vi "DPO_7K_AcquireChannels.vi"(8 "Error In":errorcluster, 10 "Settings":T3={"Channels to acquire"=[0, 1, 2, 3], "Bandwidth"=0, "#Avg"=0, "Trigger Channel"=0, "Trigger Level"=0.0, "Sampling Frequency"=0, "Epoch"=0.0, "Enable Autoscale?"=FALSE} {"Bandwidth" items=["500 MHz", "1 GHz", "2 GHz", "3 GHz", "4 GHz", "5 GHz", "6 GHz", "7 GHz", "8 GHz", "9 GHz", "10 GHz", "11 GHz", "12 GHz", "13 GHz", "14 GHz", "15 GHz", "16 GHz", "17 GHz", "18 GHz", "19 GHz", "20 GHz", "21 GHz", "22 GHz", "23 GHz", "24 GHz", "25 GHz", "26 GHz", "27 GHz", "28 GHz", "29 GHz", "30 GHz", "31 GHz", "32 GHz", "33 GHz", "33 GHz HW (Tek)", "34 GHz (ATI)", "35 GHz (ATI)", "36 GHz (ATI)", "38 GHz (ATI)", "40 GHz (ATI)", "45 GHz (ATI)", "50 GHz (ATI)"]; "Epoch" format="%#_6ps"; "Sampling Frequency" items=["3.125 Sa/s", "5 Sa/s", "6.25 Sa/s", "7.8125 Sa/s", "10 Sa/s", "12.5 Sa/s", "15.625 Sa/s", "20 Sa/s", "25 Sa/s", "31.25 Sa/s", "50 Sa/s", "62.5 Sa/s", "78.125 Sa/s", "100 Sa/s", "125 Sa/s", "156.25 Sa/s", "200 Sa/s", "250 Sa/s", "312.5 Sa/s", "390.625 Sa/s", "400 Sa/s", "500 Sa/s", "625 Sa/s", "781.25 Sa/s", "1 kSa/s", "1.25 kSa/s", "1.5625 kSa/s", "2 kSa/s", "2.5 kSa/s", "3.125 kSa/s", "3.90625 kSa/s", "4 kSa/s", "5 kSa/s", "6.25 kSa/s", "7.8125 kSa/s", "10 kSa/s", "12.5 kSa/s", "15.625 kSa/s", "20 kSa/s", "25 kSa/s", "31.25 kSa/s", "39.0625 kSa/s", "50 kSa/s", "62.5 kSa/s", "78.125 kSa/s", "100 kSa/s", "125 kSa/s", "156.25 kSa/s", "200 kSa/s", "244.14063 kSa/s", "250 kSa/s", "312.5 kSa/s", "390.625 kSa/s", "500 kSa/s", "625 kSa/s", "781.25 kSa/s", "1 MSa/s", "1.2207 MSa/s", "1.25 MSa/s", "1.5625 MSa/s", "1.95313 MSa/s", "2.44141 MSa/s", "2.5 MSa/s", "3.125 MSa/s", "3.90625 MSa/s", "4.88281 MSa/s", "5 MSa/s", "6.25 MSa/s", "7.8125 MSa/s", "9.76563 MSa/s", "12.5 MSa/s", "1.5625 MSa/s", "25 MSa/s", "31.25 MSa/s", "39.0625 MSa/s", "62.5 MSa/s", "78.125 MSa/s", "125 MSa/s", "156.25 MSa/s", "250 MSa/s", "312.5 MSa/s", "625 MSa/s", "781.25 MSa/s", "1.25 GSa/s", "1.5625 GSa/s", "3.125 GSa/s", "6.25 GSa/s", "12.5 GSa/s", "25 GSa/s", "50 GSa/s", "100 GSa/s", "200 GSa/s (ATI only)"]; "Trigger Channel" items=["Channel 1", "Channel 2", "Channel 3", "Channel 4", "Auxiliary", "Line"]; "Channels to acquire" items=["Channel 1", "Channel 2", "Channel 3", "Channel 4", "Math 1", "Math 2", "Math 3", "Math 4", "Reference 1", "Reference 2", "Reference 3", "Reference 4"]}, 11 "VISA Resource Name In":refnum<visa-resource-name>) -> (0 "Error Out":errorcluster, 2 "Acquired Data":waveform(dbl)[](array[waveform]), 3 "VISA Resource Name Out":refnum<visa-resource-name>)   [LabVIEW 2020]
uses:
  DPO 7k Settings.ctl
  subVI/Return_To_Interface.ctl
  subVI/Set_Configuration.ctl
panel:
  out "Stop":bool
  in  "Set":T1
  in  "Return to Interface":T2
  # "ACQUIRE CHANNELS"
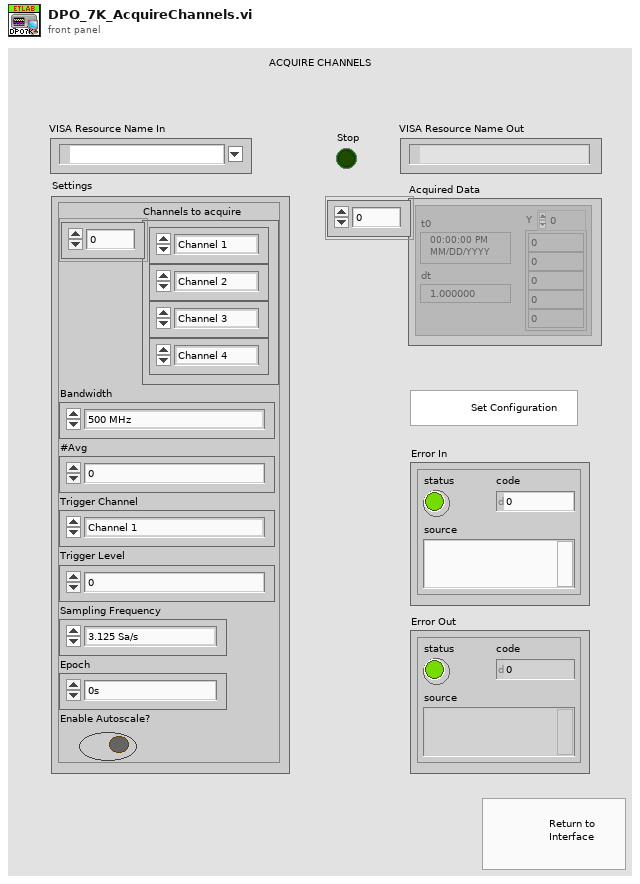
[diagram p1: front panel]
types:
  T1 = typedef "Set_Configuration.ctl" = bool
  T2 = typedef "Return_To_Interface.ctl" = bool
  T3 = typedef "DPO 7k Settings.ctl" = cluster{"Channels to acquire":u16[], "Bandwidth":u16, "#Avg":i32, "Trigger Channel":u16, "Trigger Level":dbl, "Sampling Frequency":u16, "Epoch":dbl, "Enable Autoscale?":bool}
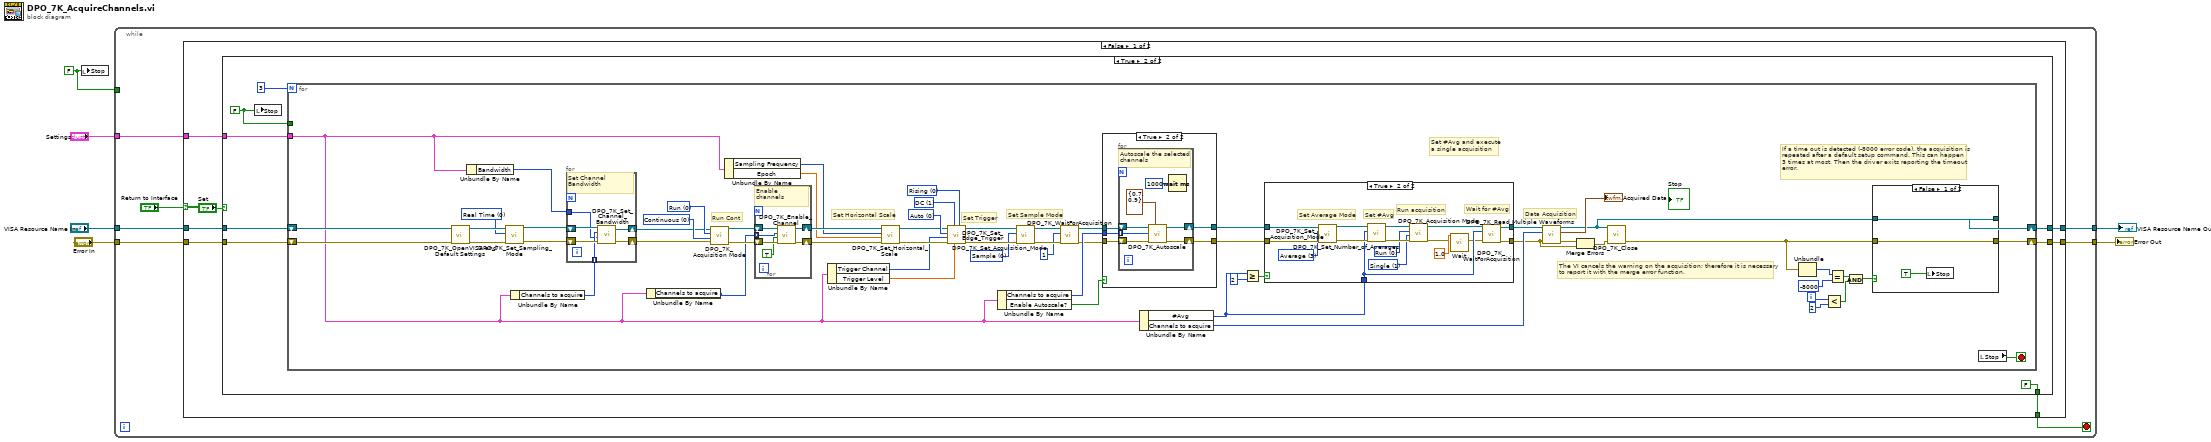
[diagram p0: block diagram]
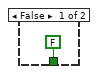
[diagram p2: hidden frame]
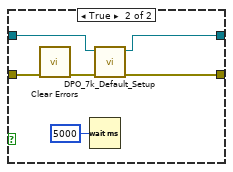
[diagram p3: hidden frame]
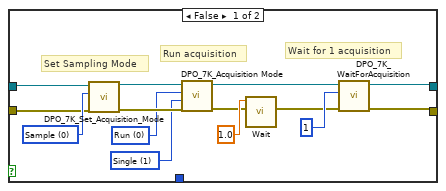
[diagram p4: hidden frame]
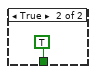
[diagram p6: hidden frame]
diagram:
  w1 = FALSE ("Stop")
  n1 = local write "Stop"(w1) -> ()
  n2 = while {
    tunnel: "Settings" -> [w9]
    tunnel: "VISA Resource Name In" -> [w12]
    tunnel: [w10] -> w3
    tunnel: "Error In" -> [w13]
    tunnel: [w11] -> w4
    tunnel: w1 -> [_]
    stop <- w7 stop-if-true
    n3 = case shown="False" "Return to Interface" {
      tunnel: w13 -> [w20 _]
      tunnel: w12 -> [w19 _]
      tunnel: [w18 _] -> w11
      tunnel: [w17 _] -> w10
      tunnel: w9 -> [w16 _]
      tunnel: [w14 TRUE] -> w7
      frame False {
        n4 = case shown="True" "Set" {
          tunnel: w20 -> [_ w29]
          tunnel: w19 -> [_ w28]
          tunnel: [_ w27] -> w18
          tunnel: [_ w26] -> w17
          tunnel: w16 -> [_ w25]
          tunnel: [FALSE FALSE] -> w14
          frame False {
          }
          frame True {
            w23 = FALSE
            n5 = local write "Stop"(w23) -> ()
            n6 = for {
              N: 3 -> [_]
              tunnel: w25 -> [w88]
              shift-right: [w86] -> w27
              shift-left: w29 -> [w90]
              shift-right: [w85] -> w26
              shift-left: w28 -> [w89]
              tunnel: w23 -> [_]
              i -> [w87]
              stop <- w30 stop-if-true
              w64 = u16 0 items=["Real Time", "Equivalent Time", "Interpolation"] ("Sampling Mode")
              w67 = u16 0 items=["Continuous", "Single"] ("Mode")
              w68 = u16 0 items=["Run", "Stop"] ("Action")
              w74 = u16 0 items=["Sample", "Peak Detect", "High resolution", "Average", "WFMDB", "Envelope"] ("Acquisition Mode")
              w82 = u16 0 items=["Auto", "Normal"] ("Trigger Mode")
              w83 = u16 1 items=["AC", "DC", "HF Reject (>50 kHz)", "LF Reject (<80 kHz)", "Noise Reject"] ("Trigger Coupling")
              w84 = u16 0 items=["Rising", "Falling", "Either"] ("Trigger Slope")
              # "If a time out is detected (-8000 error code), the acquisition is\nrepeated after a default setup command. This can happen\n3 times at most. Then the driver exits reporting the timeout\nerror."
              # "The VI cancels the warning on the acquisition; therefore it is necessary\nto report it with the merge error function."
              # "Set #Avg and execute\na single acquisition"
              # "Run Cont"
              # "Data Acquisition"
              # "Set Sample Mode"
              # "Set Trigger"
              # "Set Horizontal Scale"
              n7 = call "DPO_7K_OpenVISA and Default Settings.vi"("Error In"=w90, "VISA resource name in"=w89) -> ("error out"=w65:errorcluster, "VISA resource name out"=w66:refnum<visa-resource-name>)  [unwired: 8 in]
              n8 = Unbundle By Name(w88) -> ("Bandwidth"=w59:u16)
              n9 = call "DPO_7K_Set_Sampling_Mode.vi"("Error In"=w65, "Sampling Mode"=w64, "VISA resource name in"=w66) -> ("Error Out"=w62:errorcluster, "VISA resource name out"=w63:refnum<visa-resource-name>)  [unwired: 7 in]
              n10 = Unbundle By Name(w88) -> ("Channels to acquire"=w56:u16[])
              n11 = for {
                shift-right: [w146] -> w60
                shift-left: w63 -> [w149]
                shift-right: [w147] -> w61
                shift-left: w62 -> [w148]
                tunnel: w56 -> [w145] mode=indexing
                tunnel: w59 -> [w144]
                # "Set Channel Bandwidth"
                n12 = call "DPO_7K_Set_Channel_Bandwidth.vi"("Error In"=w148, "Bandwidth"=w144, "Channel"=w145, "VISA resource name in"=w149) -> ("Error Out"=w147:errorcluster, "VISA resource name out"=w146:refnum<visa-resource-name>)  [unwired: 6 in]
              }
              n13 = Unbundle By Name(w88) -> ("Channels to acquire"=w53:u16[])
              n14 = call "DPO_7K_Acquisition Mode.vi"("Error In"=w61, "Mode"=w67, "Action"=w68, "VISA resource name in"=w60) -> ("Error Out"=w70:errorcluster, "VISA resource name out"=w69:refnum<visa-resource-name>)  [unwired: 6 in]
              n15 = Unbundle By Name(w88) -> ("Sampling Frequency"=w58:u16, "Epoch"=w57:dbl)
              n16 = for {
                shift-right: [w154] -> w77
                shift-left: w70 -> [w153]
                shift-right: [w155] -> w78
                shift-left: w69 -> [w152]
                tunnel: w53 -> [w151] mode=indexing
                # "Enable\nchannels"
                n17 = call "DPO_7K_Enable_Channel.vi"("Error In"=w153, "Activate?"=TRUE, "Channel"=w151, "VISA resource name in"=w152) -> ("Error Out"=w154:errorcluster, "VISA resource name out"=w155:refnum<visa-resource-name>)  [unwired: 5 in, 1 out]
              }
              n18 = Unbundle By Name(w88) -> ("Trigger Channel"=w54:u16, "Trigger Level"=w55:dbl)
              n19 = call "DPO_7K_Set_Horizontal_Scale.vi"("Error In"=w77, "Epoch"=w57, "Sampling Frequency"=w58, "VISA resource name in"=w78) -> ("Error Out"=w80:errorcluster, "VISA resource name out"=w79:refnum<visa-resource-name>)  [unwired: 6 in]
              n20 = call "DPO_7K_Set_Edge_Trigger.vi"("Trigger Slope"=w84, "Trigger Level"=w55, "Trigger Coupling"=w83, "Error In"=w80, "Trigger Channel"=w54, "Trigger Mode"=w82, "VISA resource name in"=w79) -> ("Error Out"=w75:errorcluster, "VISA resource name out"=w76:refnum<visa-resource-name>)  [unwired: 3 in]
              n21 = Unbundle By Name(w88) -> ("Channels to acquire"=w52:u16[], "Enable Autoscale?"=w50:bool)
              n22 = call "DPO_7K_Set_Acquisition_Mode.vi"("Error In"=w75, "Acquisition Mode"=w74, "VISA resource name in"=w76) -> ("Error Out"=w42:errorcluster, "VISA resource name out"=w43:refnum<visa-resource-name>)  [unwired: 7 in]
              n23 = call "DPO_7K_WaitForAcquisition.vi"("Error In"=w42, "Number of Waveforms"=1, "VISA resource name in"=w43) -> ("Error Out"=w41:errorcluster, "VISA resource name out"=w40:refnum<visa-resource-name>)  [unwired: 7 in]
              n24 = case shown="True" w50 {
                tunnel: w40 -> [w131 w136]
                tunnel: w41 -> [w130 w135]
                tunnel: [w131 w134] -> w73
                tunnel: [w130 w133] -> w72
                tunnel: w52 -> [_ w132]
                frame False {
                }
                frame True {
                  n25 = for {
                    shift-right: [w141] -> w133
                    shift-left: w135 -> [w142]
                    shift-right: [w140] -> w134
                    shift-left: w136 -> [w143]
                    tunnel: w132 -> [w139] mode=indexing
                    # "Autoscale the selected channels"
                    n26 = call "DPO_7K_Autoscale.vi"("Thresholds"=cluster{"Lower":dbl, "Upper":dbl} {"Lower"=0.7, "Upper"=0.9}, "Error In"=w142, "Channel"=w139, "VISA resource name in"=w143) -> ("Error Out"=w141:errorcluster, "VISA resource name out"=w140:refnum<visa-resource-name>)  [unwired: 6 in]
                    n27 = Wait (ms)(milliseconds to wait=u32 1000) -> ()  [unwired: 1 out]
                  }
                }
              }
              n28 = Unbundle By Name(w88) -> ("#Avg"=w48:i32, "Channels to acquire"=w51:u16[])
              n29 = Greater Or Equal?(x=w48, y=2) -> (x >= y?=w49:bool)
              n30 = case shown="True" w49 {
                tunnel: [w105 w116] -> w81
                tunnel: [w106 w119] -> w45
                tunnel: w73 -> [w112 w129]
                tunnel: w72 -> [w111 w128]
                tunnel: w48 -> [_ w118]
                frame False {
                  w107 = u16 1 items=["Continuous", "Single"] ("Mode")
                  w108 = u16 0 items=["Run", "Stop"] ("Action")
                  w113 = u16 0 items=["Sample", "Peak Detect", "High resolution", "Average", "WFMDB", "Envelope"] ("Acquisition Mode")
                  # "Wait for 1 acquisition"
                  # "Run acquisition"
                  # "Set Sampling Mode"
                  n31 = call "DPO_7K_Set_Acquisition_Mode.vi"("Error In"=w111, "Acquisition Mode"=w113, "VISA resource name in"=w112) -> ("Error Out"=w109:errorcluster, "VISA resource name out"=w110:refnum<visa-resource-name>)  [unwired: 7 in]
                  n32 = call "DPO_7K_Acquisition Mode.vi"("Error In"=w109, "Mode"=w107, "Action"=w108, "VISA resource name in"=w110) -> ("Error Out"=w100:errorcluster, "VISA resource name out"=w102:refnum<visa-resource-name>)  [unwired: 6 in]
                  n33 = call "Wait.vi"("Error In"=w100, "Seconds"=1.0) -> ("Error Out"=w101:errorcluster)  [unwired: 9 in]
                  n34 = call "DPO_7K_WaitForAcquisition.vi"("Error In"=w101, "Number of Waveforms"=1, "VISA resource name in"=w102) -> ("Error Out"=w106:errorcluster, "VISA resource name out"=w105:refnum<visa-resource-name>)  [unwired: 7 in]
                }
                frame True {
                  w121 = u16 1 items=["Continuous", "Single"] ("Mode")
                  w122 = u16 0 items=["Run", "Stop"] ("Action")
                  w127 = u16 3 items=["Sample", "Peak Detect", "High resolution", "Average", "WFMDB", "Envelope"] ("Acquisition Mode")
                  # "Wait for #Avg"
                  # "Run acquisition"
                  # "Set #Avg"
                  # "Set Average Mode"
                  n35 = call "DPO_7K_Set_Acquisition_Mode.vi"("Error In"=w128, "Acquisition Mode"=w127, "VISA resource name in"=w129) -> ("Error Out"=w125:errorcluster, "VISA resource name out"=w126:refnum<visa-resource-name>)  [unwired: 7 in]
                  n36 = call "DPO_7K_Set_Number_of_Averages.vi"("Error In"=w125, "Number of Waveforms"=w118, "VISA resource name in"=w126) -> ("Error Out"=w123:errorcluster, "VISA resource name out"=w124:refnum<visa-resource-name>)  [unwired: 7 in]
                  n37 = call "DPO_7K_Acquisition Mode.vi"("Error In"=w123, "Mode"=w121, "Action"=w122, "VISA resource name in"=w124) -> ("Error Out"=w115:errorcluster, "VISA resource name out"=w117:refnum<visa-resource-name>)  [unwired: 6 in]
                  n38 = call "Wait.vi"("Error In"=w115, "Seconds"=1.0) -> ("Error Out"=w114:errorcluster)  [unwired: 9 in]
                  n39 = call "DPO_7K_WaitForAcquisition.vi"("Error In"=w114, "Number of Waveforms"=w118, "VISA resource name in"=w117) -> ("Error Out"=w119:errorcluster, "VISA resource name out"=w116:refnum<visa-resource-name>)  [unwired: 7 in]
                }
              }
              n40 = call "DPO_7K_Read Multiple Waveforms.vi"("error in (no error)"=w45, "Channels"=w51, "VISA resource name"=w81) -> ("error out"=w44:errorcluster, "Waveform Data"=→"Acquired Data":waveform(dbl)[], "VISA resource name out"=w32:refnum<visa-resource-name>)  [unwired: 5 in, 1 out]
              n41 = Merge Errors(w44, w45) -> (w46:errorcluster)
              n42 = call "DPO_7K_Close.vi"("error in (no error)"=w46, "VISA resource name"=w32) -> ("error out"=w33:errorcluster)  [unwired: 9 in]
              n43 = Unbundle(w33) -> ("code"=w38:i32)  [unwired: 2 out]
              n44 = Less?(x=w87, y=2) -> (x < y?=w35:bool)
              n45 = Equal?(x=w38, y=-8000) -> (x = y?=w36:bool)
              n46 = And(x=w36, y=w35) -> (x .and. y?=w31:bool)
              n47 = case shown="False" w31 {
                tunnel: w33 -> [w92 w99]
                tunnel: [w92 w96] -> w86
                tunnel: w32 -> [w93 w95]
                tunnel: [w93 w94] -> w85
                frame False {
                  n48 = local write "Stop"(TRUE) -> ()
                }
                frame True {
                  n49 = call <vilib>:"Clear Errors.vi"("error in (no error)"=w99) -> ("error out"=w97:errorcluster)  [unwired: 5 in, 1 out]
                  n50 = Wait (ms)(milliseconds to wait=u32 5000) -> ()  [unwired: 1 out]
                  n51 = call "DPO_7k_Default_Setup.vi"("Error in"=w97, "VISA resource name in"=w95) -> ("Error out"=w96:errorcluster, "VISA resource name out"=w94:refnum<visa-resource-name>)  [unwired: 8 in]
                }
              }
              n52 = local read "Stop"() -> (w30:bool)
            }
          }
        }
      }
      frame True {
      }
    }
  }
  "Error Out" <- w4
  "VISA Resource Name Out" <- w3
